vi "clean duplicated node mappings.vi"(8 "error in (no error)":errorcluster, 10 "Old Node":T1, 11 "New Node":T1) -> (0 "error out":errorcluster, 1 "New Engines":refnum<data-value>[](array[refnum]), 3 "New Node":T1)   [LabVIEW 2013, in "Standard Editor.lvlib"]
uses:
  Standard Editor.lvlib
  <vilib>/NI/Configuration Framework/Node/NodeRef.ctl
  <vilib>/NI/Configuration Framework/Node/NISE_CEF_Node.lvclass
  <vilib>/NI/Configuration Framework/serializable node/NISE_CEF_serializable node.lvclass
  <vilib>/NI/Configuration Framework/Node/NISE_CEF_Node.lvclass/NISE_CEF_Node.ctl
  <vilib>/NI/Configuration Framework/Node/ReadChildren.vi
  Framework Configuration Classes/class cache/cache data.vi
  <vilib>/NI/Configuration Framework/serializable configuration/NISE_CEF_serializable configuration.lvclass
  Framework Configuration Classes/class cache/PL_class cache.lvlib
panel:
  out "Engine":bool
  out "Target":bool
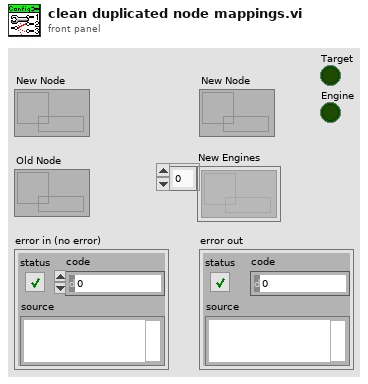
[diagram p1: front panel]
types:
  T1 = typedef "NISE_CEF_Node.lvclass/NodeRef.ctl" = refnum<data-value>
  T2 = typedef "PL_class cache.lvlib/cached class information.ctl" = cluster{"targets":T3[], "engines":T4[], "modules":T4[], "ignored class list":path[]}
  T3 = typedef "PL_class cache.lvlib/target class metadata.ctl" = cluster{"file name":string, "fully qualified name":string, "menu display name":string, "configuration class name":string}
  T4 = typedef "PL_class cache.lvlib/class metadata.ctl" = cluster{"file name":string, "fully qualified name":string, "menu display name":string, "configuration class":string, "category":string, "instances allowed":i32, "supported targets":T5[]}
  T5 = typedef "TBM configuration.lvclass/Target Types.ctl" = enum16{"Windows", "Mac", "Linux", "Linux RT ARM", "VxWorks", "Pharlap", "Other", "Linux RT x64"}
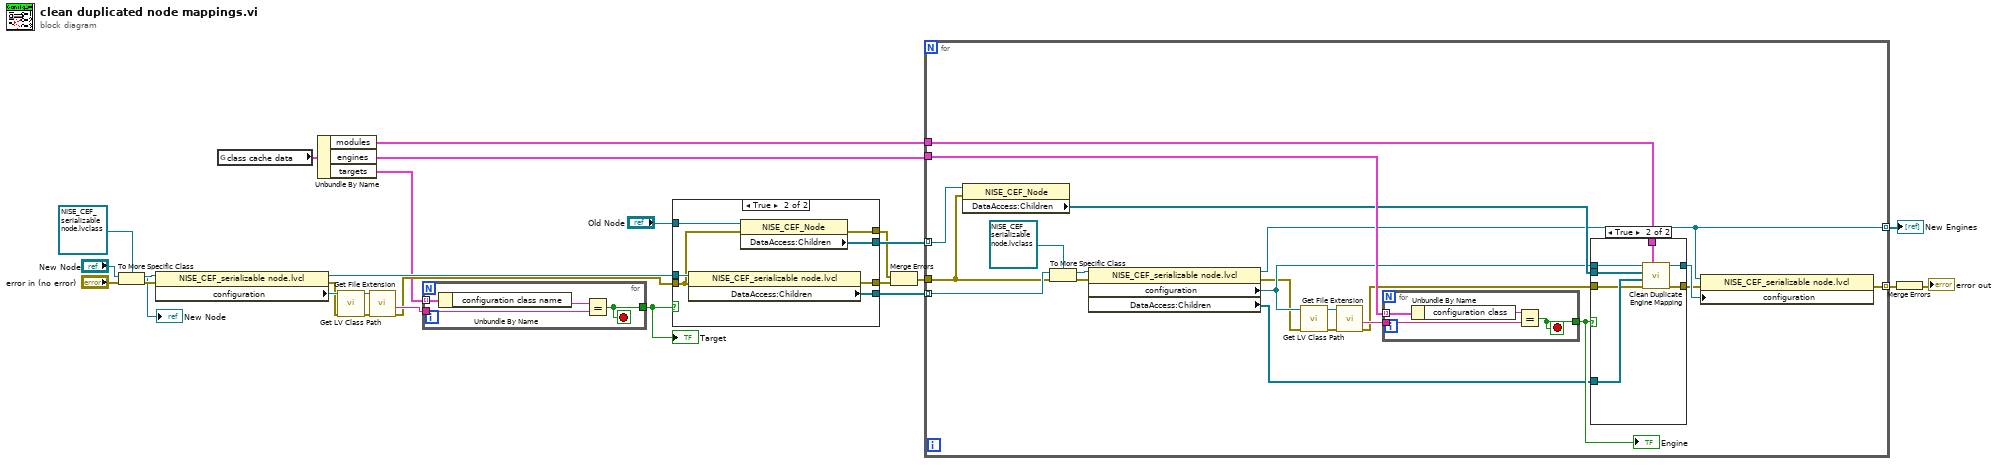
[diagram p0: block diagram]
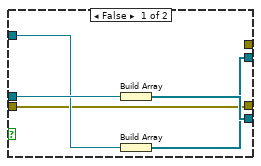
[diagram p3: hidden frame]
diagram:
  n1 = To More Specific Class(target class=refnum<data-value> refnum, reference="New Node", error in="error in (no error)") -> (specific class reference=w25:refnum<data-value>, error out=w24:errorcluster)
  n2 = property class="NISE_CEF_serializable node.lvcl"(reference=w25, error in=w24) -> (reference out=w17:refnum<data-value>, error out=w9:errorcluster, "configuration"=w20:refnum<class "NISE_CEF_serializable configuration.lvclass">)
  n3 = global read "cache data.vi" "class cache data"() -> (w22:T2)
  n4 = Unbundle By Name(w22) -> ("modules"=w2:T4[], "engines"=w3:T4[], "targets"=w4:T3[])
  n5 = call <vilib>:"Get LV Class Path.vi"("error in (no error)"=w9, "object"=w20) -> ("error out"=w8:errorcluster, "class path"=w23:path)  [unwired: 8 in]
  n6 = call <vilib>:"Get File Extension.vi"("error in (no error)"=w8, "file"=w23) -> ("error out"=w7:errorcluster, "filename without extension"=w21:string)  [unwired: 6 in, 2 out]
  n7 = for {
    tunnel: w4 -> [w30] mode=indexing
    tunnel: w21 -> [w28]
    tunnel: [w27] -> w19
    stop <- w27 stop-if-true
    n8 = Unbundle By Name(w30) -> ("configuration class name"=w29:string)
    n9 = Equal?(x=w29, y=w28) -> (x = y?=w27:bool)
  }
  "Target" <- w19
  n10 = case shown="True" w19 {
    tunnel: w17 -> [w35 w42]
    tunnel: [w34 w41] -> w16
    tunnel: "Old Node" -> [w33 w40]
    tunnel: [w32 w39] -> w14
    tunnel: [_ w38] -> w12
    tunnel: [w31 w37] -> w11
    tunnel: w7 -> [w31 w36]
    frame False {
      n11 = Build Array(w35) -> (w34:refnum<data-value>[])
      n12 = Build Array(w33) -> (w32:T1[])
    }
    frame True {
      n13 = property class="NISE_CEF_serializable node.lvcl"(reference=w42, error in=w36) -> (error out=w37:errorcluster, "DataAccess:Children"=w41:T1[])  [unwired: 1 out]
      n14 = property class="NISE_CEF_Node"(reference=w40, error in=w36) -> (error out=w38:errorcluster, "DataAccess:Children"=w39:T1[])  [unwired: 1 out]
    }
  }
  n15 = Merge Errors(w12, w11) -> (w13:errorcluster)
  n16 = for {
    tunnel: w3 -> [w63]
    tunnel: w2 -> [w61]
    tunnel: w16 -> [w52] mode=indexing
    tunnel: w14 -> [w53] mode=indexing
    tunnel: w13 -> [w48]
    tunnel: [w47] -> w5 mode=indexing
    tunnel: [w43] -> w1 mode=indexing
    n17 = property class="NISE_CEF_Node"(reference=w53, error in=w48) -> ("DataAccess:Children"=w58:T1[])  [unwired: 2 out]
    n18 = To More Specific Class(target class=refnum<data-value> refnum, reference=w52, error in=w48) -> (specific class reference=w51:refnum<data-value>, error out=w49:errorcluster)
    n19 = property class="NISE_CEF_serializable node.lvcl"(reference=w51, error in=w49) -> (reference out=w43:refnum<data-value>, error out=w45:errorcluster, "configuration"=w57:refnum<class "NISE_CEF_serializable configuration.lvclass">, "DataAccess:Children"=w54:T1[])
    n20 = call <vilib>:"Get LV Class Path.vi"("error in (no error)"=w45, "object"=w57) -> ("error out"=w46:errorcluster, "class path"=w56:path)  [unwired: 8 in]
    n21 = call <vilib>:"Get File Extension.vi"("error in (no error)"=w46, "file"=w56) -> ("error out"=w44:errorcluster, "filename without extension"=w55:string)  [unwired: 6 in, 2 out]
    n22 = for {
      tunnel: w63 -> [w76] mode=indexing
      tunnel: w55 -> [w74]
      tunnel: [w73] -> w62
      stop <- w73 stop-if-true
      n23 = Unbundle By Name(w76) -> ("configuration class"=w75:string)
      n24 = Equal?(x=w75, y=w74) -> (x = y?=w73:bool)
    }
    "Engine" <- w62
    n25 = case shown="True" w62 {
      tunnel: w57 -> [w65 w70]
      tunnel: w54 -> [_ w72]
      tunnel: w58 -> [_ w71]
      tunnel: w61 -> [_ w66]
      tunnel: [w65 w69] -> w60
      tunnel: w44 -> [w64 w68]
      tunnel: [w64 w67] -> w59
      frame False {
      }
      frame True {
        n26 = call "Clean Duplicate Engine Mapping.vi"("modules"=w66, "error in (no error)"=w68, "New Children"=w72, "Old Children"=w71, "Engine configuration in"=w70) -> ("error out"=w67:errorcluster, "Engine configuration out"=w69:refnum<class "NISE_CEF_serializable configuration.lvclass">)  [unwired: 5 in]
      }
    }
    n27 = property class="NISE_CEF_serializable node.lvcl"(reference=w43, error in=w59, "configuration"=w60) -> (error out=w47:errorcluster)  [unwired: 1 out]
  }
  "New Engines" <- w1
  n28 = Merge Errors(w5) -> (→"error out":errorcluster)
  "New Node" <- "New Node"
